vi "Update Time.vi"(8 "error in (no error)":errorcluster, 11 "Time in":u64) -> (0 "error out":errorcluster, 3 "Time out":u64)   [LabVIEW 2021, in "ChannelCommon.lvlib"]
uses:
  ChannelCommon.lvlib
  CIFUtilities/CIFClocks/CIFClocks.lvlib
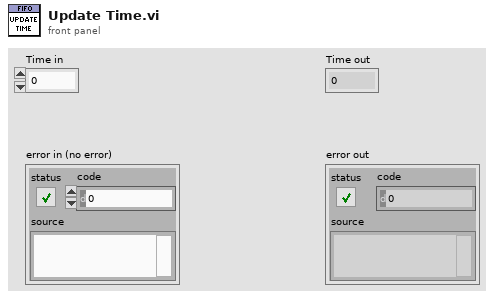
[diagram p1: front panel]
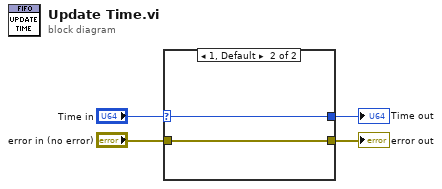
[diagram p0: block diagram]
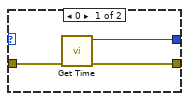
[diagram p2: hidden frame]
diagram:
  n1 = case shown="1, Default" "Time in" {
    selector: "Time in" -> [_ w9]
    tunnel: [w5 w9] -> w3
    tunnel: "error in (no error)" -> [w7 w8]
    tunnel: [w6 w8] -> w1
    frame 0 {
      n2 = call "Get Time.vi"("error in (no error)"=w7) -> ("error out"=w6:errorcluster, "Time (ns)"=w5:u64)  [unwired: 8 in, 1 out]
    }
    frame 1, Default {
    }
  }
  "Time out" <- w3
  "error out" <- w1
